vi "Write Table Custom infos.vi"(0 "PDF Table Class.lvclass in":refnum<class "Pdfp Table Class.lvclass">, 1 "Font et paragraph":T10, 2 "Table type":T11, 3 "Row Header?":bool, 5 "Repeat Headers Row":bool=TRUE, 7 "Table columnWidth [ ]":sgl[](array[numeric]), 9 "Header Column size":cluster{"# Column":u16, "# Row":u16}, 11 "error in (no error)":errorcluster, 12 "Table size":cluster{"# Column":u16, "# Row":u16}, 13 "Text Table 2D [ ]":string[][](array[string]), 14 "Image to Add [ ]":T12 {"Scale" format="%#_g %"}) -> (4 "PDF Table Class.lvclass out":refnum<class "Pdfp Table Class.lvclass">, 15 "error out":errorcluster)   [LabVIEW 2019, in "Pdfp Table Class.lvclass"]
uses:
  <userlib>/Exaprom PDF/LV Class/Pdfp Table Class/Pdfp Table Class.lvclass
  <userlib>/Exaprom PDF/Controls/General Controls/Image to Add [ ].ctl
  <userlib>/Exaprom PDF/Controls/Image Controls/Image Scale.ctl
  <userlib>/Exaprom PDF/Controls/Table Controls/Table type.ctl
  <userlib>/Exaprom PDF/Controls/Initialization Controls/Defaut Paragraphe and Line Spacing.ctl
  <userlib>/Exaprom PDF/Controls/Text Controls/Texte alignement.ctl
  <userlib>/Exaprom PDF/Controls/Text Controls/Line spacing.ctl
  <userlib>/Exaprom PDF/Controls/Font Controls/Font complete cluster.ctl
  <userlib>/Exaprom PDF/Controls/Font Controls/Font size.ctl
  <userlib>/Exaprom PDF/Controls/Font Controls/Font color.ctl
  <userlib>/Exaprom PDF/Controls/Font Controls/Type and encoding.ctl
  <userlib>/Exaprom PDF/Controls/Text Controls/Unicode/Type and run direction.ctl
  C:/Program Files/National Instruments/LabVIEW 2019/user.lib/Exaprom PDF/DLL/itextsharp.dll
  DLL/itextsharp.dll
  <userlib>/Exaprom PDF/Controls/Font Controls/System Fonts.ctl
  <userlib>/Exaprom PDF/LV Class/Pdfp Table Class/Pdfp Table Class.lvclass/Pdfp Table Class.ctl
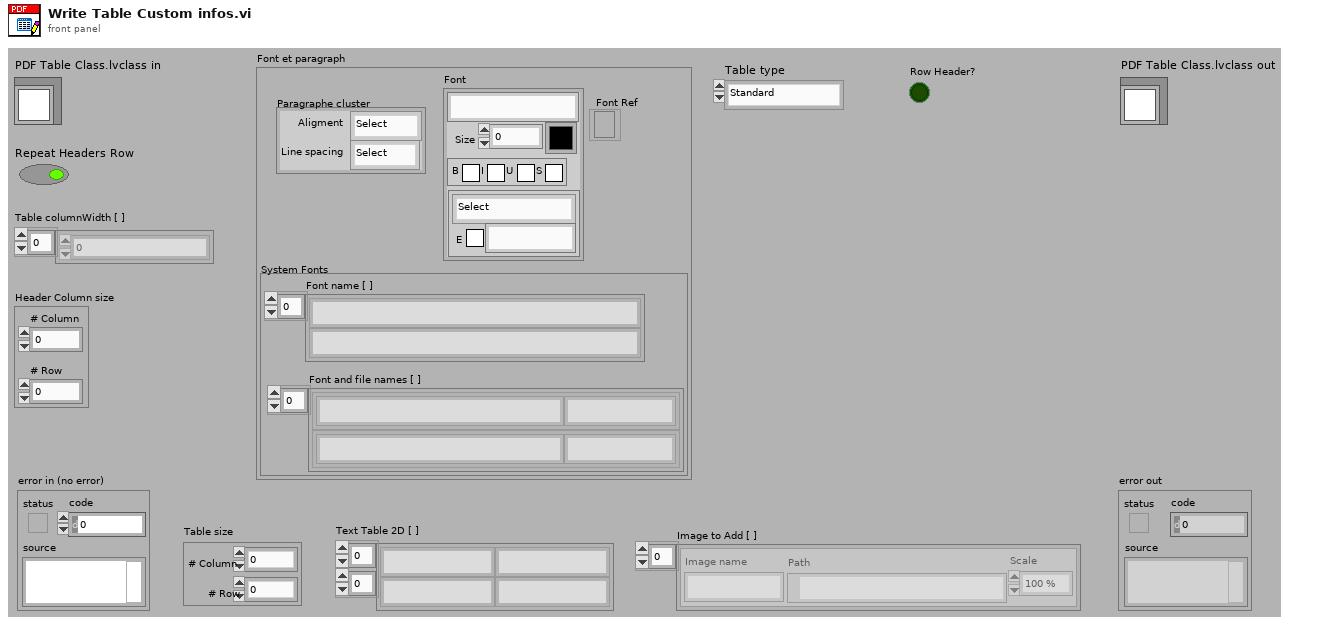
[diagram p1: front panel]
types:
  T1 = typedef "Defaut Paragraphe and Line Spacing.ctl" = cluster{" Aligment":T2, "Line spacing":T3}
  T2 = typedef "Texte alignement.ctl" = enum16{"Select", "CENTER", "JUSTIFY", "LEFT", "RIGHT"}
  T3 = typedef "Line spacing.ctl" = enum16{"Select", "1.0", "1.5", "2.0"}
  T4 = typedef "Font complete cluster.ctl" = cluster{"Name":string, "Size":T5, "Color":T6, "Style":cluster{"Bold":bool, "Italic":bool, "Underline":bool, "Strikeout":bool}, "Type":T7}
  T5 = typedef "Font size.ctl" = sgl
  T6 = typedef "Font color.ctl" = u32
  T7 = typedef "Type and encoding.ctl" = cluster{"Type&direction":T8, "Embedded":bool, "Encoding":string}
  T8 = typedef "Type and run direction.ctl" = enum16{"Select", "ASCII", "UTF-16", "UTF-16 (default)", "UTF-16 (LTR)", "UTF-16 (RTL)"}
  T9 = typedef "System Fonts.ctl" = cluster{"Font name [ ]":string[], "Font and file names [ ]":cluster{"Font name":string, "File name":string}[]}
  T10 = cluster{"Paragraphe cluster":T1, "Font":T4, "Font Ref":refnum<k24>, "System Fonts":T9}
  T11 = typedef "Table type.ctl" = enum16{"Standard", "Customized"}
  T12 = typedef "Image to Add [ ].ctl" = cluster{"Image name":string, "Path":path, "Scale":T13}[]
  T13 = typedef "Image Scale.ctl" = sgl
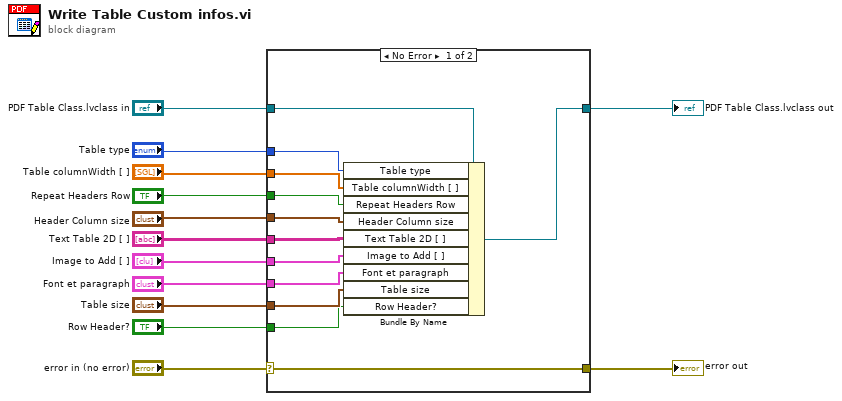
[diagram p0: block diagram]
diagram:
  n1 = case shown="No Error" "error in (no error)" {
    selector: "error in (no error)" -> [w25 w26]
    tunnel: [w25 w26] -> w12
    tunnel: [w23 w27] -> w10
    tunnel: "PDF Table Class.lvclass in" -> [w24 w27]
    tunnel: "Repeat Headers Row" -> [w22 _]
    tunnel: "Table type" -> [w21 _]
    tunnel: "Table columnWidth [ ]" -> [w20 _]
    tunnel: "Header Column size" -> [w19 _]
    tunnel: "Text Table 2D [ ]" -> [w18 _]
    tunnel: "Image to Add [ ]" -> [w17 _]
    tunnel: "Font et paragraph" -> [w16 _]
    tunnel: "Table size" -> [w15 _]
    tunnel: "Row Header?" -> [w14 _]
    frame No Error {
      n2 = Bundle By Name(cluster=w24, "Table type"=w21, "Table columnWidth [ ]"=w20, "Repeat Headers Row"=w22, "Header Column size"=w19, "Text Table 2D [ ]"=w18, "Image to Add [ ]"=w17, "Font et paragraph"=w16, "Table size"=w15, "Row Header?"=w14) -> (w23:refnum<class "Pdfp Table Class.lvclass">)
    }
    frame Error {
    }
  }
  "error out" <- w12
  "PDF Table Class.lvclass out" <- w10
